vi "Parse.vi"(8 "Error In":errorcluster, 11 "object in":refnum<class "2021_9.lvclass">) -> (0 "Error Out":errorcluster, 3 "object out":refnum<class "2021_9.lvclass">)   [LabVIEW 2020, in "2021_9.lvclass"]
uses:
  2021_9.lvclass
  2021_9.lvclass/2021_9.ctl
panel:
  out "Array":i32[][](array[numeric])
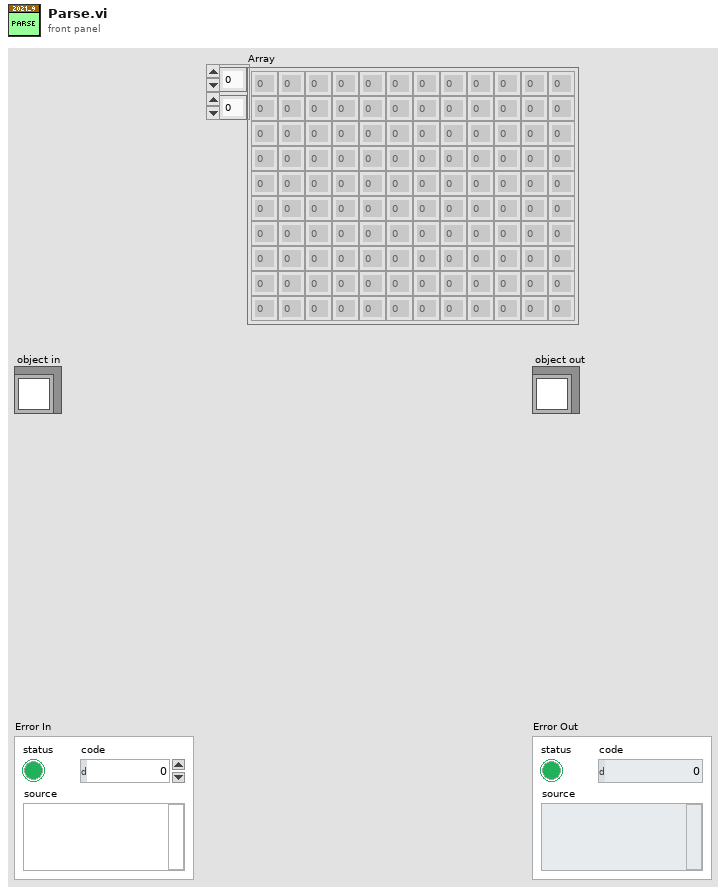
[diagram p1: front panel]
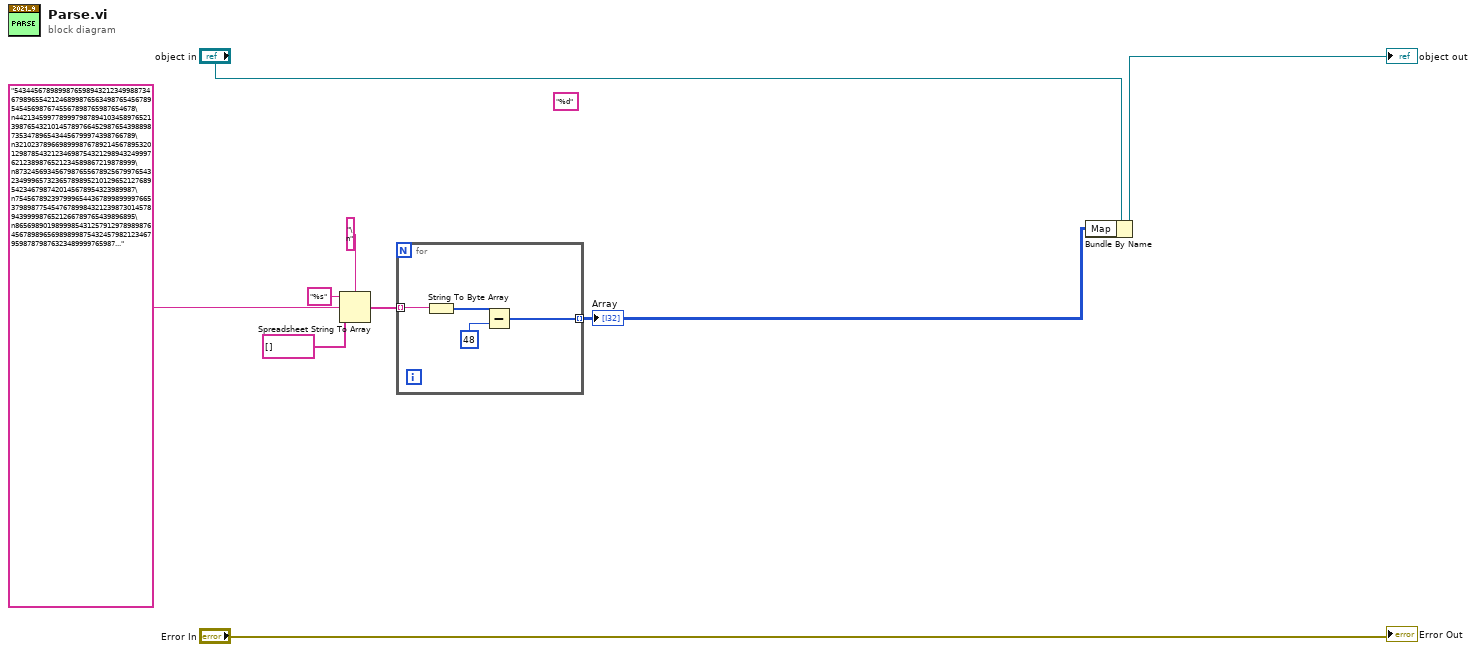
[diagram p0: block diagram]
diagram:
  (unwired) "%d" ("format string")
  n1 = Spreadsheet String To Array(delimiter (Tab)="\n", format string="%s", spreadsheet string="5434456789899876598943212349988734679896554212468998765634987654567895454569876745567898765987654678\n4421345997789997987894103458976521398765432101457897664529876543988987353478965434456799974398766789\n3210237896698999876789214567895320129878543212346987543212989432499976212389876521234589867219878999\n8732456934567987655678925679976543234999657323657898952101296521276895423467987420145678954323989987\n7545678923979996544367899899997665379898775454767899843212398730145789439999876521266789765439896895\n86569890198999854312579129789898764567898965698989987543245798212346795987879876323489999765987..." ("PuzzleInput"), array type (2D Dbl)=string[] []) -> (array=w2:string[])
  n2 = for {
    tunnel: w2 -> [w13] mode=indexing
    tunnel: [w10] -> w1 mode=indexing
    n3 = String To Byte Array(string=w13) -> (unsigned byte array=w12:u8[])
    n4 = Subtract(x=w12, y=48) -> (x-y=w10:i32[])
  }
  "Array" <- w1
  n5 = Bundle By Name(cluster="object in", "Map"=w1) -> (→"object out":refnum<class "2021_9.lvclass">)
  "Error Out" <- "Error In"
